vi "Get Path.vi"(8 "error in (no error)":errorcluster, 11 "PathMsg in":refnum<class "PathMsg.lvclass">) -> (0 "error out":errorcluster, 2 "Message Data":path, 3 "PathMsg out":refnum<class "PathMsg.lvclass">)   [LabVIEW 2013, in "LapDog.Messaging.v3.NativeTypes.lvlib" / "PathMsg.lvclass"]
doc: "Returns the data contained in the message.\n\nThis method executes regardless of the error in state."
uses:
  PathMsg.lvclass
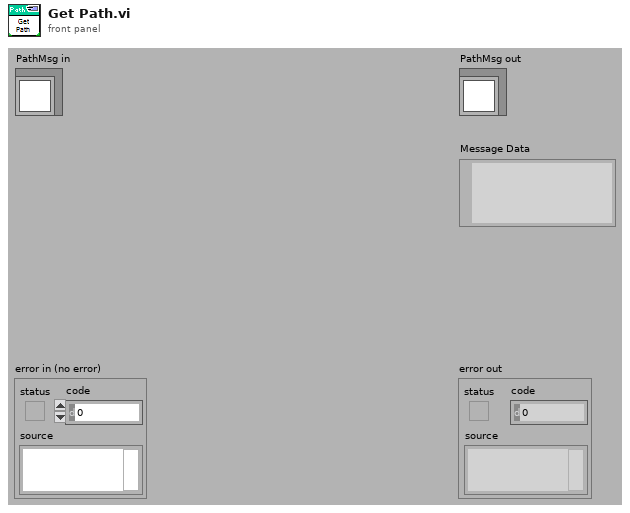
[diagram p1: front panel]
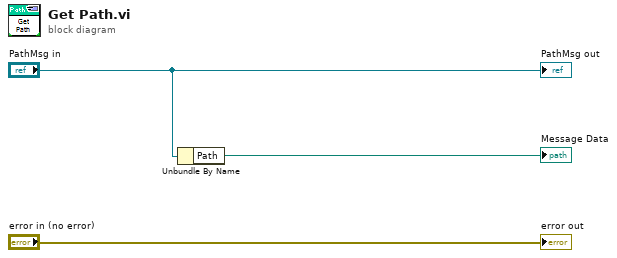
[diagram p0: block diagram]
diagram:
  n1 = Unbundle By Name("PathMsg in") -> ("Path"=→"Message Data":path)
  "error out" <- "error in (no error)"
  "PathMsg out" <- "PathMsg in"
